vi "XiXi-1(Divide U32).vi"(10 "X[-1]":u32, 11 "Xi":u32[](array[numeric])) -> (2 "Remain":u32[](array[numeric]), 3 "Yi":u32[](array[numeric]))   [LabVIEW 2012]
doc: "Calculate sums of consecutive array elements. 0th element of output is equal to x(0)+ x(-1), where x(-1) is an optional scalar input that defaults to zero."
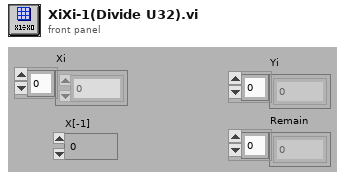
[diagram p1: front panel]
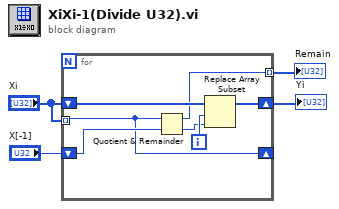
[diagram p0: block diagram]
diagram:
  n1 = for {
    shift-right: [w10] -> w2
    shift-left: "Xi" -> [w11]
    shift-right: [w6] -> _
    shift-left: "X[-1]" -> [w8]
    tunnel: "Xi" -> [w6] mode=indexing
    tunnel: [w5] -> w1 mode=indexing
    i -> [w9]
    n2 = Quotient & Remainder(x=w6, y=w8) -> (x-y*floor(x/y)=w5:u32, floor(x/y)=w7:u32)
    n3 = Replace Array Subset(array=w11, new element=w7, index=w9) -> (w10:u32[])
  }
  "Yi" <- w2
  "Remain" <- w1
